vi "DestroyObjRef.vi"(8 "error in (no error)":errorcluster, 11 "reference in":refnum<class "PSU_Base.lvclass">) -> (0 "error out":errorcluster, 3 "reference out":refnum<class "PSU_Base.lvclass">)   [LabVIEW 2022 SP3, in "PSU_Base.lvlib" / "PSU_Base.lvclass"]
uses:
  PSU_Base.lvclass
  PSU_Base.lvclass/PSU_Base.ctl
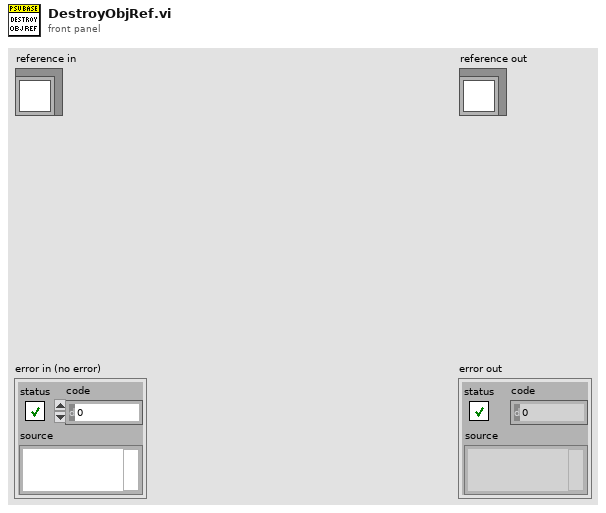
[diagram p1: front panel]
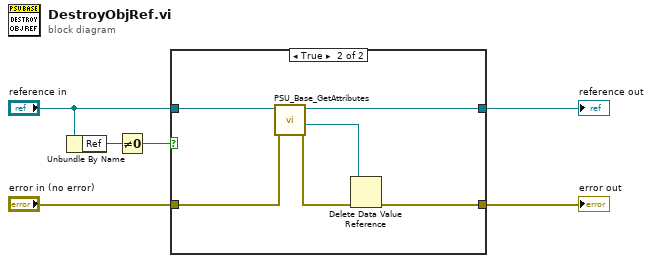
[diagram p0: block diagram]
diagram:
  n1 = Unbundle By Name("reference in") -> ("Ref"=w3:u32)
  n2 = Not Equal To 0?(x=w3) -> (x != 0?=w2:bool)
  n3 = case shown="True" w2 {
    tunnel: [w7 w11] -> w6
    tunnel: [w8 w13] -> w5
    tunnel: "reference in" -> [w8 w14]
    tunnel: "error in (no error)" -> [w7 w9]
    frame False {
    }
    frame True {
      n4 = call "PSU_Base_GetAttributes.vi"("error in (no error)"=w9, "reference in"=w14) -> ("error out"=w12:errorcluster, "DataRef"=w10:refnum<data-value>, "reference out"=w13:refnum<class "PSU_Base.lvclass">)  [unwired: 6 in, 1 out]
      n5 = Delete Data Value Reference(data value reference=w10, error in=w12) -> (error out=w11:errorcluster)  [unwired: 1 out]
    }
  }
  "error out" <- w6
  "reference out" <- w5
